vi "Teleop.vi"(0 "Call Context":T2, 1 "Match Info":T1={"Autonomous Elapsed Seconds"=0.0, "TeleOp Elapsed Seconds"=0.0, "Disabled Elapsed Seconds"=0.0, "Visited Autonomous"=FALSE, "Visited TeleOp"=FALSE, "Visited Disabled"=FALSE, "Autonomous Settings"={"Autonomous Style"=enum."Independent", "VI Refnum"=refnum}}) -> ()   [LabVIEW 2018]
doc: "This VI is called for each TeleOp packet received from the DS where the robot is not disabled. It is often used to read from the joysticks and update I/O or to update setpoints for timed control loops. It should complete and return within 20 milliseconds or it may miss DS packets."
uses:
  <vilib>/Rock Robotics/WPI/DriverStation/WPI_DriverStationDerivedRobotMode.ctl
  <vilib>/Rock Robotics/WPI/DriverStation/WPI_DriverStationMatch Info.ctl
  <vilib>/Rock Robotics/WPI/ThirdParty/Phoenix-LabVIEW/Motor Controller/Controls/CTRE_Phoenix_MotorControl_ControlMode.ctl
  <vilib>/Rock Robotics/WPI/Solenoid/WPI_SolenoidValue.ctl
  <vilib>/Rock Robotics/WPI/Utilities/WPI_GetSetVariantRefNum.vi
  <vilib>/Rock Robotics/Network Tables/NT Write Boolean Array.vi
  <vilib>/Rock Robotics/Network Tables/NT Write Numeric Array.vi
  <vilib>/Rock Robotics/Network Tables/NT Read Boolean.vi
  <vilib>/Rock Robotics/Network Tables/NT Read Number.vi
  <vilib>/Rock Robotics/WPI/Ultrasonic/WPI_SonarMB1010AnalogRefNum Registry Get.vi
  <vilib>/Rock Robotics/WPI/Ultrasonic/WPI_SonarMB1010AnalogGetRange.vi
  <vilib>/Rock Robotics/Network Tables/NT Write Number.vi
  <vilib>/Rock Robotics/WPI/Solenoid/WPI_SolenoidSetEnum.vi
panel:
  out "Distance":dbl
  out "FarRight":bool
  out "NearRight":bool
  out "NearLeft":bool
  out "FarLeft":bool
  out "Center":bool
  out "Compressor Running":bool
  out "Enabled":bool
  out "Sample Slider 0":dbl(slide) scale=0.0..5.0
  out "Sample Boolean 1":bool
  out "Sample Boolean 0":bool
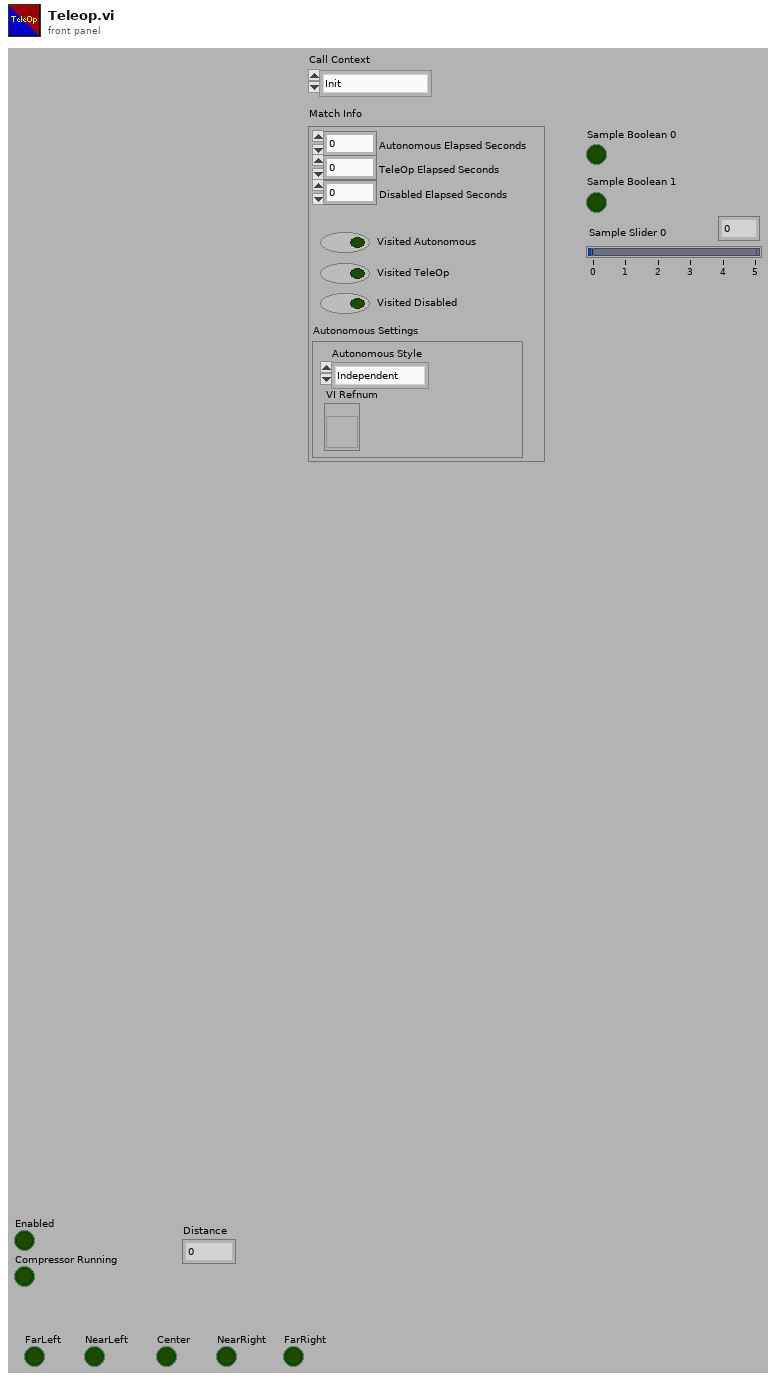
[diagram p1: front panel]
types:
  T1 = typedef "WPI_DriverStationMatch Info.ctl" = cluster{"Autonomous Elapsed Seconds":dbl, "TeleOp Elapsed Seconds":dbl, "Disabled Elapsed Seconds":dbl, "Visited Autonomous":bool, "Visited TeleOp":bool, "Visited Disabled":bool, "Autonomous Settings":cluster{"Autonomous Style":enum16{"Iterative", "Independent"}, "VI Refnum":refnum<vi>}}
  T2 = typedef "WPI_DriverStationDerivedRobotMode.ctl" = enum16{"Init", "Execute", "Stop"}
  T3 = typedef "WPI_JoystickDevRef.ctl" = cluster{"Device":T4}
  T4 = typedef "WPI_JoystickDeviceEnum.ctl" = enum16{"USB 0", "USB 1", "USB 2", "USB 3", "USB 4", "USB 5"}
  T5 = typedef "WPI_DigitalInputDevRef.ctl" = cluster{"DevStatus":errorcluster, "DIO Channel":T6}
  T6 = typedef "FPGA_DIOChannel.ctl" = enum8{"DIO 0", "DIO 1", "DIO 2", "DIO 3", "DIO 4", "DIO 5", "DIO 6", "DIO 7", "DIO 8", "DIO 9", "DIO MXP 0", "DIO MXP 1", "DIO MXP 2", "DIO MXP 3", "DIO MXP 4", "DIO MXP 5", "DIO MXP 6", "DIO MXP 7", "DIO MXP 8", "DIO MXP 9", "DIO MXP 10", "DIO MXP 11", "DIO MXP 12", "DIO MXP 13", "DIO MXP 14", "DIO MXP 15", "SPI Port CS1", "SPI Port CS2", "SPI Port CS3", "SPI Port MISO", "SPI Port MOSI", "Invalid"}
  T7 = typedef "CTRE_Phoenix_MotorControl_ControlMode.ctl" = u16
  T8 = typedef "WPI_MotorControlDeviceRef.ctl" = cluster{"DeviceStatus":errorcluster, "Type":T9, "PWM":cluster{"PWM Channel":T10, "DeadBand":T11}, "CAN":cluster{"Device Number":u8, "SetOutput VI Ref":variant, "GetOutput VI Ref":variant, "Enable VI Ref":variant, "Disable VI Ref":variant, "Data":variant}, "Invert":bool, "DIO PWM":cluster{"PWM \"Enable\" Channel":T10, "DIOChannel":T6, "PWM Rate":dbl}}
  T9 = typedef "WPI_MotorControlType.ctl" = enum16{"PWM", "CAN", "DIO PWM"}
  T10 = typedef "FPGA_DIOPWMChannel.ctl" = enum8{"PWM 0", "PWM 1", "PWM 2", "PWM 3", "PWM 4", "PWM 5", "PWM 6", "PWM 7", "PWM 8", "PWM 9", "PWM MXP 0", "PWM MXP 1", "PWM MXP 2", "PWM MXP 3", "PWM MXP 4", "PWM MXP 5", "PWM MXP 6", "PWM MXP 7", "PWM MXP 8", "PWM MXP 9", "Invalid"}
  T11 = typedef "WPI_PWMDeadband.ctl" = cluster{"Name":string, "maxPositivePwm":i32, "minPositivePwm":i32, "centerPwm":i32, "maxNegativePwm":i32, "minNegativePwm":i32, "angularRange":u16}
  T12 = typedef "WPI_SolenoidValue.ctl" = enum16{"Off", "On", "Forward", "Reverse"}
  T13 = typedef "WPI_SolenoidDevRef.ctl" = cluster{"DevStatus":errorcluster, "Pneumatics Control Module":u8, "Forward Solenoid Channel":T14, "Reverse Solenoid Channel":T14}
  T14 = typedef "WPI_SolenoidChannel.ctl" = enum8{"Solenoid 0", "Solenoid 1", "Solenoid 2", "Solenoid 3", "Solenoid 4", "Solenoid 5", "Solenoid 6", "Solenoid 7", "Invalid"}
  T15 = typedef "WPI_SonarMB1010AnalogDeviceRef.ctl" = cluster{"AIDeviceRef":T16, "Scaling factor (V/in)":dbl, "Average Bits":u8}
  T16 = typedef "WPI_AnalogChannelDevRef.ctl" = cluster{"DevStatus":errorcluster, "Analog Channel":T17}
  T17 = typedef "FPGA_AIChannel.ctl" = enum8{"AI 0", "AI 1", "AI 2", "AI 3", "AI MXP 0", "AI MXP 1", "AI MXP 2", "AI MXP 3", "Invalid"}
  T18 = typedef "WPI_CompressorDevRef.ctl" = cluster{"DevStatus":errorcluster, "Pneumatics Control Module":u8}
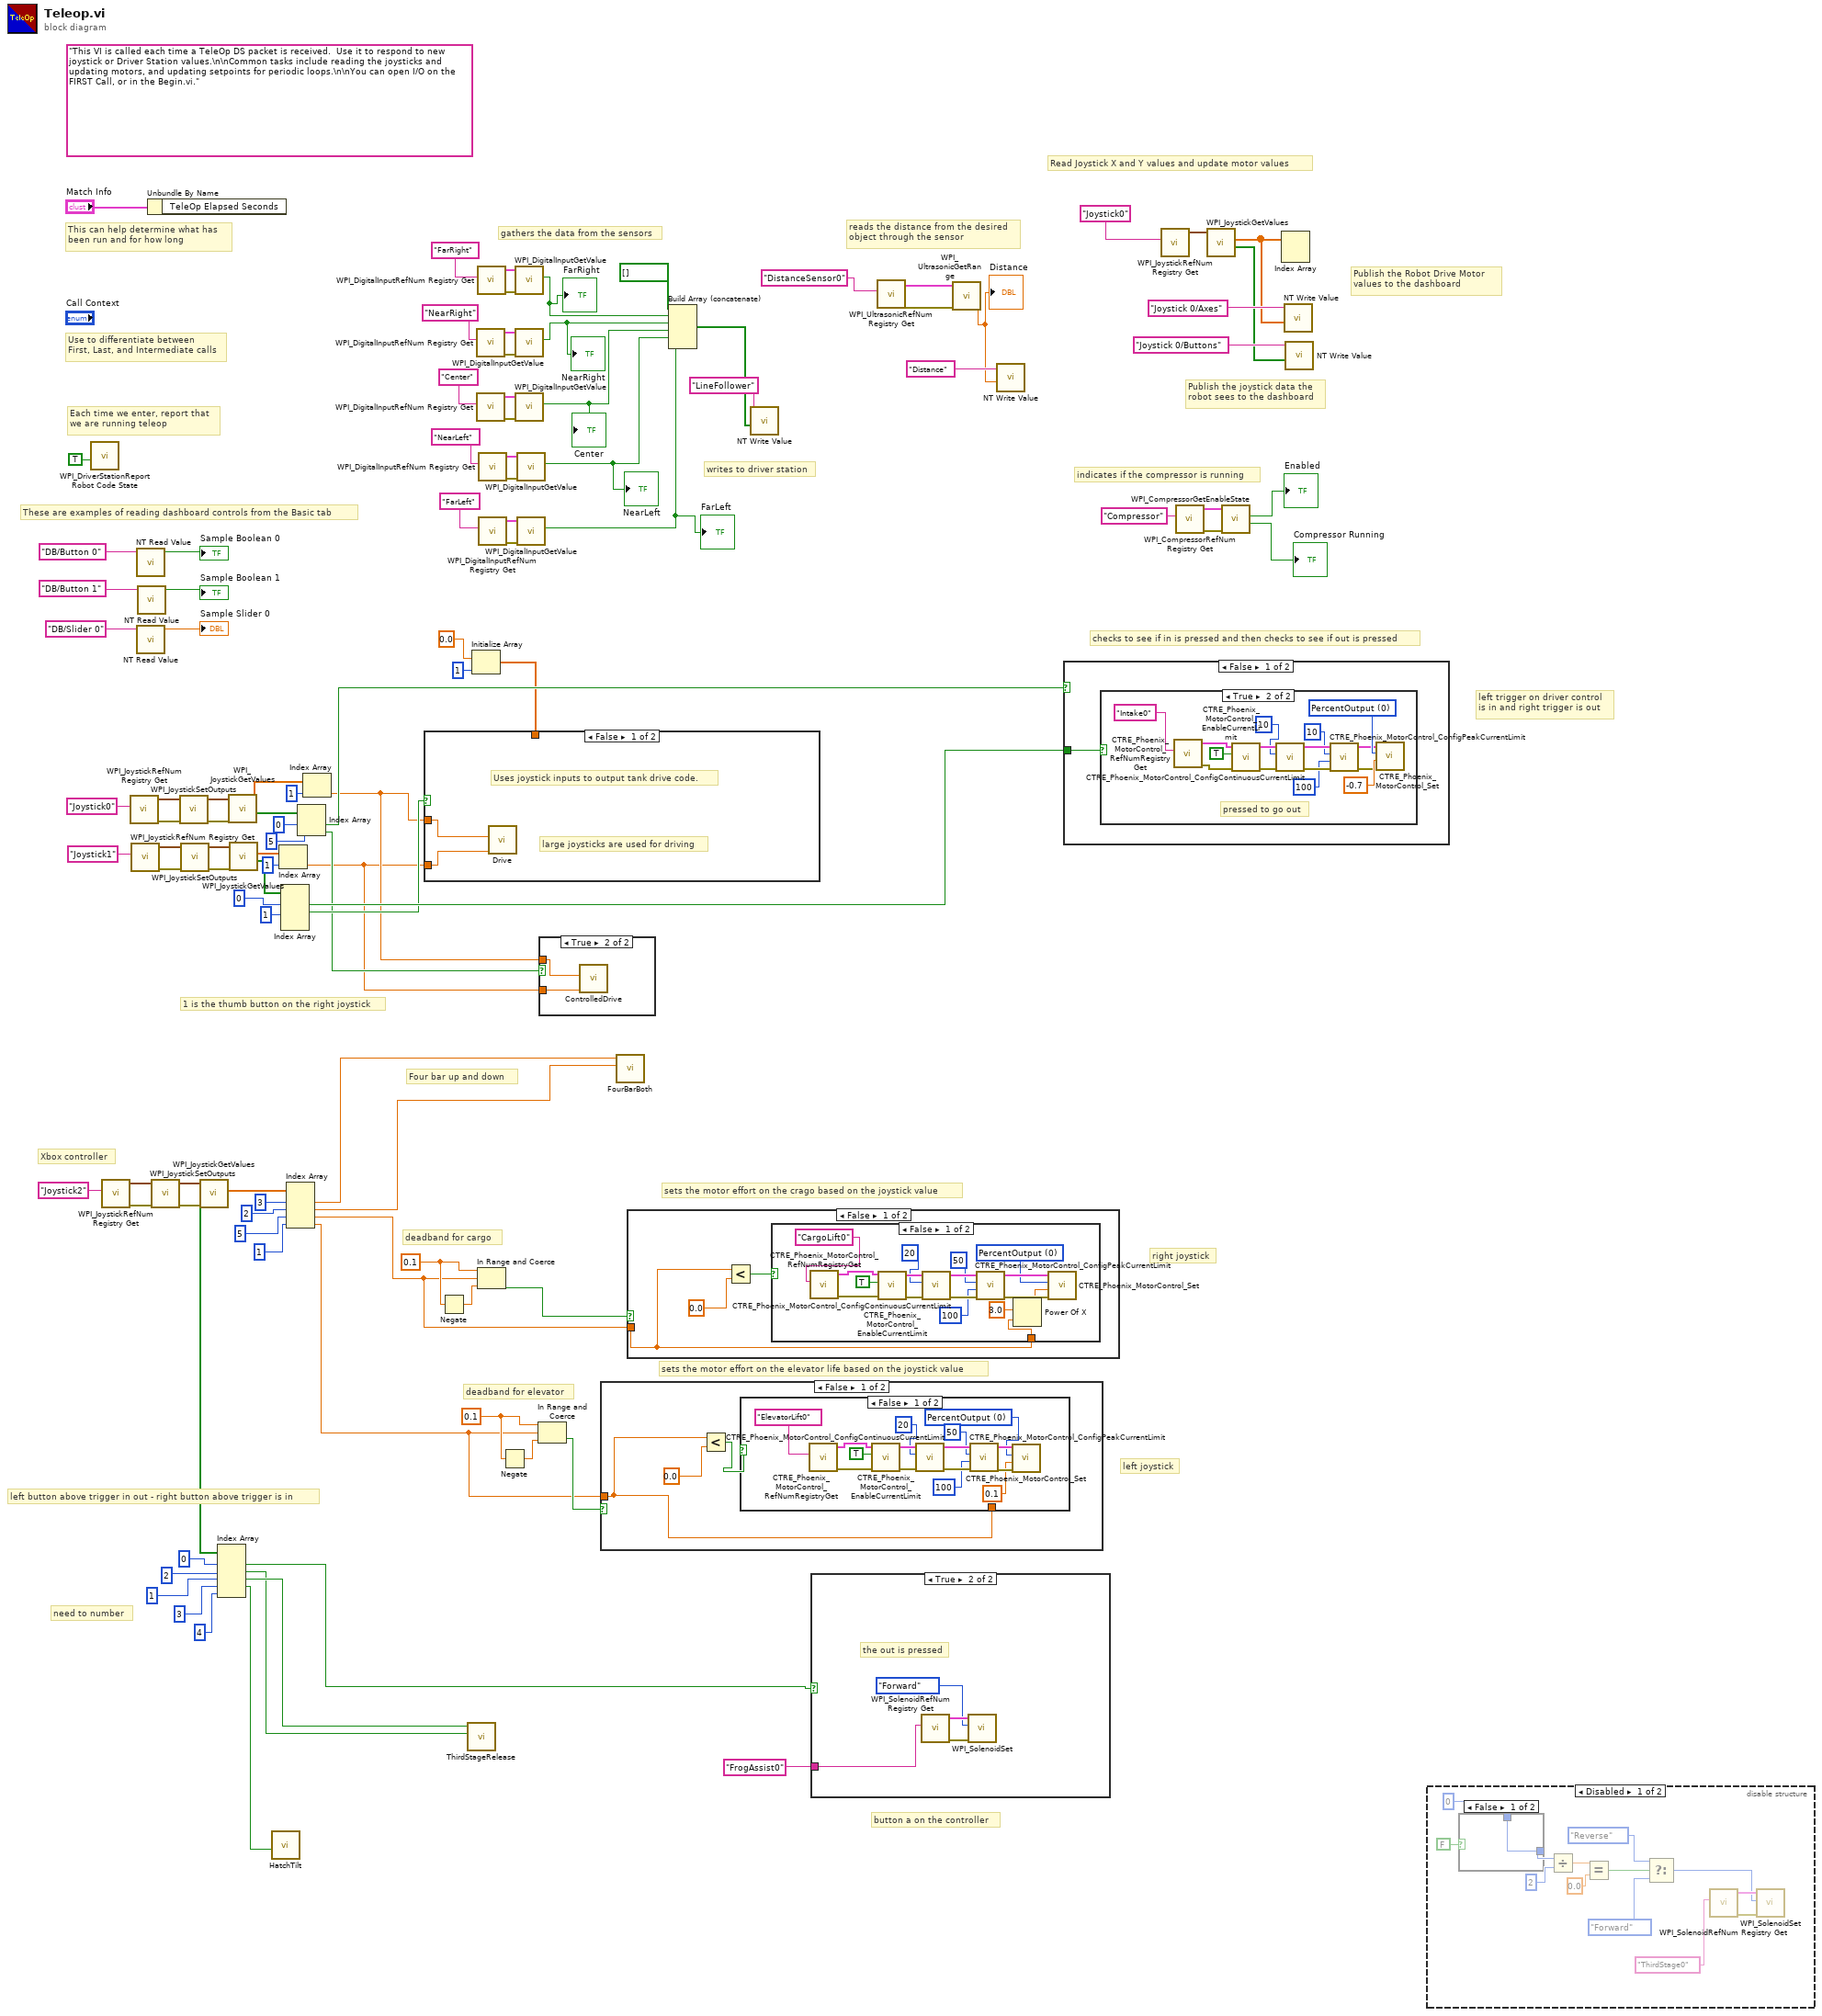
[diagram p0: block diagram]
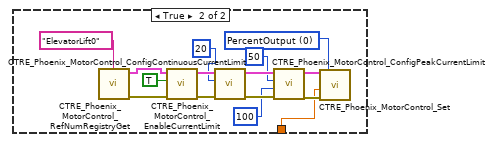
[diagram p3: hidden frame]
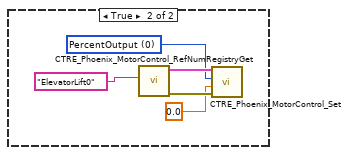
[diagram p4: hidden frame]
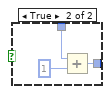
[diagram p5: hidden frame]
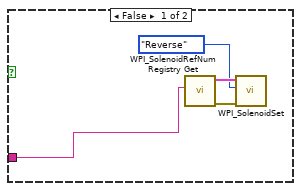
[diagram p7: hidden frame]
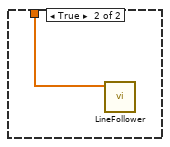
[diagram p8: hidden frame]
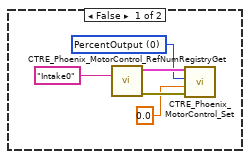
[diagram p9: hidden frame]
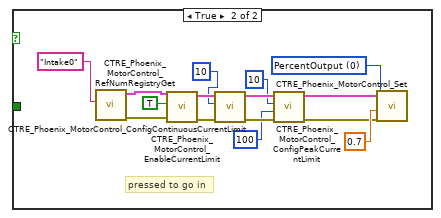
[diagram p10: hidden frame]
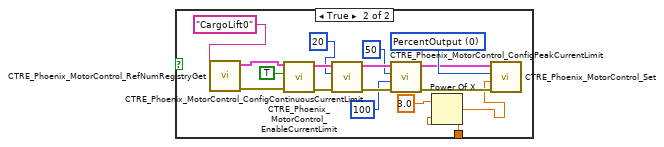
[diagram p11: hidden frame]
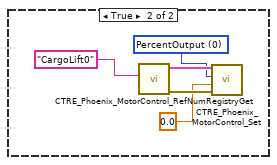
[diagram p12: hidden frame]
diagram:
  w52 = 0.1 ("upper limit")
  w55 = 0.1 ("upper limit")
  (unwired) "This VI is called each time a TeleOp DS packet is received.  Use it to respond to new joystick or Driver Station values.\n\nCommon tasks include reading the joysticks and updating motors, and updating setpoints for periodic loops.\n\nYou can open I/O on the FIRST Call, or in the Begin.vi."
  # "left joystick"
  # "sets the motor effort on the elevator life based on the joystick value"
  # "reads the distance from the desired\nobject through the sensor"
  # "button a on the controller"
  # "gathers the data from the sensors"
  # "writes to driver station"
  # "1 is the thumb button on the right joystick"
  # "left trigger on driver control\nis in and right trigger is out"
  # "checks to see if in is pressed and then checks to see if out is pressed"
  # "right joystick"
  # "deadband for elevator"
  # "deadband for cargo"
  # "sets the motor effort on the crago based on the joystick value"
  # "Four bar up and down"
  # "indicates if the compressor is running"
  # "need to number"
  # "left button above trigger in out - right button above trigger is in"
  # "Xbox controller"
  # "These are examples of reading dashboard controls from the Basic tab"
  # "Publish the Robot Drive Motor\nvalues to the dashboard"
  # "Publish the joystick data the\nrobot sees to the dashboard"
  # "Each time we enter, report that\nwe are running teleop"
  # "Use to differentiate between\nFirst, Last, and Intermediate calls"
  # "This can help determine what has\nbeen run and for how long"
  # "Read Joystick X and Y values and update motor values"
  n1 = call <vilib>:"WPI_DriverStationReport Robot Code State.vi"("TeleOp"=TRUE ("Autonomous")) -> ()  [unwired: 10 in, 1 out]
  n2 = call <vilib>:"WPI_JoystickRefNum Registry Get.vi"("refnum name"="Joystick2") -> ("error out"=w76:errorcluster, "JoystickDevRef"=w78:T3)  [unwired: 1 in, 8 out]
  n3 = call <vilib>:"WPI_JoystickRefNum Registry Get.vi"("refnum name"="Joystick0") -> ("error out"=w89:errorcluster, "JoystickDevRef"=w91:T3)  [unwired: 1 in, 8 out]
  n4 = call <vilib>:"WPI_JoystickRefNum Registry Get.vi"("refnum name"="Joystick1") -> ("error out"=w86:errorcluster, "JoystickDevRef"=w84:T3)  [unwired: 1 in, 8 out]
  n5 = call-poly <vilib>:"NT Read Value.vi"("Name"="DB/Button 0" ("refnum name")) -> ("Boolean"=→"Sample Boolean 0":bool)  [unwired: 9 in, 1 out]
  n6 = call-poly <vilib>:"NT Read Value.vi"("Name"="DB/Slider 0" ("refnum name")) -> ("Numeric"=→"Sample Slider 0":dbl)  [unwired: 9 in, 1 out]
  n7 = call-poly <vilib>:"NT Read Value.vi"("Name"="DB/Button 1" ("refnum name")) -> ("Boolean"=→"Sample Boolean 1":bool)  [unwired: 9 in, 1 out]
  n8 = Unbundle By Name("Match Info") -> ()  [unwired: 1 out]
  n9 = call <vilib>:"WPI_JoystickSetOutputs.vi"("error in (no error)"=w76, "JoystickDevRef"=w78) -> ("error out"=w75:errorcluster, "JoystickDevRef"=w77:T3)  [unwired: 8 in]
  n10 = call <vilib>:"WPI_JoystickSetOutputs.vi"("error in (no error)"=w89, "JoystickDevRef"=w91) -> ("error out"=w88:errorcluster, "JoystickDevRef"=w90:T3)  [unwired: 8 in]
  n11 = call <vilib>:"WPI_JoystickSetOutputs.vi"("error in (no error)"=w86, "JoystickDevRef"=w84) -> ("error out"=w87:errorcluster, "JoystickDevRef"=w85:T3)  [unwired: 8 in]
  n12 = call <vilib>:"WPI_JoystickGetValues.vi"("error in (no error)"=w75, "JoystickDevRef"=w77) -> ("Buttons"=w74:bool[], "Axes"=w71:dbl[])  [unwired: 5 in, 3 out]
  n13 = Index Array(array=w74, index #1=0 ("index"), index #2=2 ("index"), index #3=1 ("index"), index #4=3 ("index"), index #5=4 ("index")) -> (element #1=w16:bool, element #2=w8:bool, element #3=w9:bool, element #4=w10:bool)  [unwired: 1 out]
  n14 = call <vilib>:"WPI_JoystickGetValues.vi"("error in (no error)"=w88, "JoystickDevRef"=w90) -> ("Buttons"=w80:bool[], "Axes"=w93:dbl[])  [unwired: 5 in, 3 out]
  n15 = call <vilib>:"WPI_JoystickGetValues.vi"("error in (no error)"=w87, "JoystickDevRef"=w85) -> ("Buttons"=w65:bool[], "Axes"=w82:dbl[])  [unwired: 5 in, 3 out]
  n16 = call "HatchTilt.vi"("Boolean"=w10) -> ()  [unwired: 11 in]
  n17 = Index Array(array=w82, index=1) -> (element=w1:dbl)
  n18 = Index Array(array=w65, index #1=0 ("index"), index #2=1 ("index")) -> (element #1=w46:bool, element #2=w21:bool)  [unwired: 2 in, 2 out]
  n19 = Index Array(array=w71, index #1=3 ("index"), index #2=2 ("index"), index #3=5 ("index"), index #4=1 ("index")) -> (element #1=w6:dbl, element #2=w5:dbl, element #3=w54:dbl, element #4=w50:dbl)
  n20 = Index Array(array=w80, index #1=0 ("index"), index #2=5 ("index")) -> (element #1=w47:bool, element #2=w3:bool)
  n21 = Index Array(array=w93, index=1) -> (element=w2:dbl)
  n22 = Negate(x=w55) -> (-x=w57:dbl)
  n23 = call "ThirdStageRelease.vi"("In"=w8, "Out"=w9) -> ()  [unwired: 10 in]
  n24 = Initialize Array(0.0 ("element"), 1 ("dimension size")) -> (w18:dbl[])
  n25 = case shown="False" w21 {
    tunnel: w2 -> [w109 _]
    tunnel: w1 -> [w108 _]
    tunnel: w18 -> [_ w110]
    frame False {
      # "large joysticks are used for driving"
      # "Uses joystick inputs to output tank drive code."
      n26 = call "Drive.vi"("Drive R"=w108, "Drive L"=w109) -> ()  [unwired: 10 in]
    }
    frame True {
      n27 = call "LineFollower.vi"("LastNumArray"=w110) -> ()  [unwired: 11 in]
    }
  }
  n28 = call <vilib>:"WPI_DigitalInputRefNum Registry Get.vi"("refnum name"="NearRight") -> ("error out"=w41:errorcluster, "DigitalInputDevRef"=w40:T5)  [unwired: 9 in]
  n29 = call <vilib>:"WPI_DigitalInputRefNum Registry Get.vi"("refnum name"="Center") -> ("error out"=w38:errorcluster, "DigitalInputDevRef"=w37:T5)  [unwired: 9 in]
  n30 = call <vilib>:"WPI_DigitalInputRefNum Registry Get.vi"("refnum name"="FarRight") -> ("error out"=w44:errorcluster, "DigitalInputDevRef"=w43:T5)  [unwired: 9 in]
  n31 = In Range and Coerce(upper limit=w55, x=w54, lower limit=w57) -> (In Range?=w56:bool)  [unwired: 1 out]
  n32 = call <vilib>:"WPI_DigitalInputRefNum Registry Get.vi"("refnum name"="NearLeft") -> ("error out"=w35:errorcluster, "DigitalInputDevRef"=w34:T5)  [unwired: 9 in]
  n33 = call <vilib>:"WPI_DigitalInputRefNum Registry Get.vi"("refnum name"="FarLeft") -> ("error out"=w32:errorcluster, "DigitalInputDevRef"=w31:T5)  [unwired: 9 in]
  n34 = Negate(x=w52) -> (-x=w53:dbl)
  n35 = call <vilib>:"WPI_DigitalInputGetValue.vi"("error in (no error)"=w44, "DigitalInputDevRef"=w43) -> ("Value"=w28:bool)  [unwired: 7 in, 2 out]
  "FarRight" <- w28
  n36 = call <vilib>:"WPI_DigitalInputGetValue.vi"("error in (no error)"=w41, "DigitalInputDevRef"=w40) -> ("Value"=w27:bool)  [unwired: 7 in, 2 out]
  "NearRight" <- w27
  n37 = call <vilib>:"WPI_DigitalInputGetValue.vi"("error in (no error)"=w38, "DigitalInputDevRef"=w37) -> ("Value"=w29:bool)  [unwired: 7 in, 2 out]
  "Center" <- w29
  n38 = call <vilib>:"WPI_DigitalInputGetValue.vi"("error in (no error)"=w35, "DigitalInputDevRef"=w34) -> ("Value"=w26:bool)  [unwired: 7 in, 2 out]
  "NearLeft" <- w26
  n39 = call <vilib>:"WPI_DigitalInputGetValue.vi"("error in (no error)"=w32, "DigitalInputDevRef"=w31) -> ("Value"=w25:bool)  [unwired: 7 in, 2 out]
  "FarLeft" <- w25
  n40 = In Range and Coerce(upper limit=w52, x=w50, lower limit=w53) -> (In Range?=w51:bool)  [unwired: 1 out]
  n41 = case shown="True" w3 {
    tunnel: w2 -> [_ w112]
    tunnel: w1 -> [_ w111]
    frame False {
    }
    frame True {
      n42 = call "ControlledDrive.vi"("Drive R"=w111, "Drive L"=w112) -> ()  [unwired: 10 in]
    }
  }
  n43 = case shown="False" w51 {
    tunnel: w50 -> [w113 _]
    frame False {
      n44 = Less?(x=w113, y=0.0) -> (x < y?=w115:bool)
      n45 = case shown="False" w115 {
        tunnel: w113 -> [_ w131]
        frame False {
          w122 = T7 0 items=["PercentOutput"=0, "Position"=1, "Velocity"=2, "Current"=3, "Follower"=5, "MotionProfile"=6, "MotionMagic"=7, "MotionMagicArc"=8, "MotionProfileArc"=10, "Disabled"=15] ("Control Mode")
          n46 = call <vilib>:"CTRE_Phoenix_MotorControl_RefNumRegistryGet.vi"("refnum name"="ElevatorLift0") -> ("error out"=w128:errorcluster, "PhoenixMotorControlDevRef"=w127:T8)  [unwired: 9 in]
          n47 = call <vilib>:"CTRE_Phoenix_MotorControl_EnableCurrentLimit.vi"("error in (no error)"=w128, "Enable Current Limit?"=TRUE, "PhoenixMotorControlDevRef"=w127) -> ("error out"=w123:errorcluster, "PhoenixMotorControlDevRef"=w124:T8)  [unwired: 7 in]
          n48 = call <vilib>:"CTRE_Phoenix_MotorControl_ConfigContinuousCurrentLimit.vi"("error in (no error)"=w123, "Continuous Current Limit (Amps)"=20, "PhoenixMotorControlDevRef"=w124) -> ("error out"=w126:errorcluster, "PhoenixMotorControlDevRef"=w125:T8)  [unwired: 7 in]
          n49 = call <vilib>:"CTRE_Phoenix_MotorControl_ConfigPeakCurrentLimit.vi"("error in (no error)"=w126, "Peak Current Maximum Duration (ms)"=100, "Peak Current (Amps)"=50, "PhoenixMotorControlDevRef"=w125) -> ("error out"=w130:errorcluster, "PhoenixMotorControlDevRef"=w129:T8)  [unwired: 6 in]
          n50 = call <vilib>:"CTRE_Phoenix_MotorControl_Set.vi"("error in (no error)"=w130, "Output"=0.1, "Control Mode"=w122, "PhoenixMotorControlDevRef"=w129) -> ()  [unwired: 6 in, 2 out]
        }
        frame True {
          w145 = T7 0 items=["PercentOutput"=0, "Position"=1, "Velocity"=2, "Current"=3, "Follower"=5, "MotionProfile"=6, "MotionMagic"=7, "MotionMagicArc"=8, "MotionProfileArc"=10, "Disabled"=15] ("Control Mode")
          n51 = call <vilib>:"CTRE_Phoenix_MotorControl_RefNumRegistryGet.vi"("refnum name"="ElevatorLift0") -> ("error out"=w135:errorcluster, "PhoenixMotorControlDevRef"=w136:T8)  [unwired: 9 in]
          n52 = call <vilib>:"CTRE_Phoenix_MotorControl_EnableCurrentLimit.vi"("error in (no error)"=w135, "Enable Current Limit?"=TRUE, "PhoenixMotorControlDevRef"=w136) -> ("error out"=w142:errorcluster, "PhoenixMotorControlDevRef"=w141:T8)  [unwired: 7 in]
          n53 = call <vilib>:"CTRE_Phoenix_MotorControl_ConfigContinuousCurrentLimit.vi"("error in (no error)"=w142, "Continuous Current Limit (Amps)"=20, "PhoenixMotorControlDevRef"=w141) -> ("error out"=w139:errorcluster, "PhoenixMotorControlDevRef"=w140:T8)  [unwired: 7 in]
          n54 = call <vilib>:"CTRE_Phoenix_MotorControl_ConfigPeakCurrentLimit.vi"("error in (no error)"=w139, "Peak Current Maximum Duration (ms)"=100, "Peak Current (Amps)"=50, "PhoenixMotorControlDevRef"=w140) -> ("error out"=w133:errorcluster, "PhoenixMotorControlDevRef"=w134:T8)  [unwired: 6 in]
          n55 = call <vilib>:"CTRE_Phoenix_MotorControl_Set.vi"("error in (no error)"=w133, "Output"=w131, "Control Mode"=w145, "PhoenixMotorControlDevRef"=w134) -> ()  [unwired: 6 in, 2 out]
        }
      }
    }
    frame True {
      w146 = T7 0 items=["PercentOutput"=0, "Position"=1, "Velocity"=2, "Current"=3, "Follower"=5, "MotionProfile"=6, "MotionMagic"=7, "MotionMagicArc"=8, "MotionProfileArc"=10, "Disabled"=15] ("Control Mode")
      n56 = call <vilib>:"CTRE_Phoenix_MotorControl_RefNumRegistryGet.vi"("refnum name"="ElevatorLift0") -> ("error out"=w150:errorcluster, "PhoenixMotorControlDevRef"=w149:T8)  [unwired: 9 in]
      n57 = call <vilib>:"CTRE_Phoenix_MotorControl_Set.vi"("error in (no error)"=w150, "Output"=0.0, "Control Mode"=w146, "PhoenixMotorControlDevRef"=w149) -> ()  [unwired: 6 in, 2 out]
    }
  }
  n58 = call "FourBarBoth.vi"("Down"=w5, "Up"=w6) -> ()  [unwired: 10 in]
  n59 = case shown="False" w56 {
    tunnel: w54 -> [w151 _]
    frame False {
      n60 = Less?(x=w151, y=0.0) -> (x < y?=w152:bool)
      n61 = case shown="False" w152 {
        tunnel: w151 -> [w155 w171]
        frame False {
          w162 = T7 0 items=["PercentOutput"=0, "Position"=1, "Velocity"=2, "Current"=3, "Follower"=5, "MotionProfile"=6, "MotionMagic"=7, "MotionMagicArc"=8, "MotionProfileArc"=10, "Disabled"=15] ("Control Mode")
          n62 = call <vilib>:"CTRE_Phoenix_MotorControl_RefNumRegistryGet.vi"("refnum name"="CargoLift0") -> ("error out"=w168:errorcluster, "PhoenixMotorControlDevRef"=w167:T8)  [unwired: 9 in]
          n63 = call <vilib>:"CTRE_Phoenix_MotorControl_EnableCurrentLimit.vi"("error in (no error)"=w168, "Enable Current Limit?"=TRUE, "PhoenixMotorControlDevRef"=w167) -> ("error out"=w163:errorcluster, "PhoenixMotorControlDevRef"=w164:T8)  [unwired: 7 in]
          n64 = call <vilib>:"CTRE_Phoenix_MotorControl_ConfigContinuousCurrentLimit.vi"("error in (no error)"=w163, "Continuous Current Limit (Amps)"=20, "PhoenixMotorControlDevRef"=w164) -> ("error out"=w166:errorcluster, "PhoenixMotorControlDevRef"=w165:T8)  [unwired: 7 in]
          n65 = call <vilib>:"CTRE_Phoenix_MotorControl_ConfigPeakCurrentLimit.vi"("error in (no error)"=w166, "Peak Current Maximum Duration (ms)"=100, "Peak Current (Amps)"=50, "PhoenixMotorControlDevRef"=w165) -> ("error out"=w170:errorcluster, "PhoenixMotorControlDevRef"=w169:T8)  [unwired: 6 in]
          n66 = Power Of X(1:w155, 2:3.0 ("y")) -> (0:w154:dbl)
          n67 = call <vilib>:"CTRE_Phoenix_MotorControl_Set.vi"("error in (no error)"=w170, "Output"=w154, "Control Mode"=w162, "PhoenixMotorControlDevRef"=w169) -> ()  [unwired: 6 in, 2 out]
        }
        frame True {
          w187 = T7 0 items=["PercentOutput"=0, "Position"=1, "Velocity"=2, "Current"=3, "Follower"=5, "MotionProfile"=6, "MotionMagic"=7, "MotionMagicArc"=8, "MotionProfileArc"=10, "Disabled"=15] ("Control Mode")
          n68 = call <vilib>:"CTRE_Phoenix_MotorControl_RefNumRegistryGet.vi"("refnum name"="CargoLift0") -> ("error out"=w178:errorcluster, "PhoenixMotorControlDevRef"=w179:T8)  [unwired: 9 in]
          n69 = call <vilib>:"CTRE_Phoenix_MotorControl_EnableCurrentLimit.vi"("error in (no error)"=w178, "Enable Current Limit?"=TRUE, "PhoenixMotorControlDevRef"=w179) -> ("error out"=w185:errorcluster, "PhoenixMotorControlDevRef"=w184:T8)  [unwired: 7 in]
          n70 = call <vilib>:"CTRE_Phoenix_MotorControl_ConfigContinuousCurrentLimit.vi"("error in (no error)"=w185, "Continuous Current Limit (Amps)"=20, "PhoenixMotorControlDevRef"=w184) -> ("error out"=w182:errorcluster, "PhoenixMotorControlDevRef"=w183:T8)  [unwired: 7 in]
          n71 = call <vilib>:"CTRE_Phoenix_MotorControl_ConfigPeakCurrentLimit.vi"("error in (no error)"=w182, "Peak Current Maximum Duration (ms)"=100, "Peak Current (Amps)"=50, "PhoenixMotorControlDevRef"=w183) -> ("error out"=w176:errorcluster, "PhoenixMotorControlDevRef"=w177:T8)  [unwired: 6 in]
          n72 = Power Of X(1:w171, 2:3.0 ("y")) -> (0:w173:dbl)
          n73 = call <vilib>:"CTRE_Phoenix_MotorControl_Set.vi"("error in (no error)"=w176, "Output"=w173, "Control Mode"=w187, "PhoenixMotorControlDevRef"=w177) -> ()  [unwired: 6 in, 2 out]
        }
      }
    }
    frame True {
      w189 = T7 0 items=["PercentOutput"=0, "Position"=1, "Velocity"=2, "Current"=3, "Follower"=5, "MotionProfile"=6, "MotionMagic"=7, "MotionMagicArc"=8, "MotionProfileArc"=10, "Disabled"=15] ("Control Mode")
      n74 = call <vilib>:"CTRE_Phoenix_MotorControl_RefNumRegistryGet.vi"("refnum name"="CargoLift0") -> ("error out"=w192:errorcluster, "PhoenixMotorControlDevRef"=w191:T8)  [unwired: 9 in]
      n75 = call <vilib>:"CTRE_Phoenix_MotorControl_Set.vi"("error in (no error)"=w192, "Output"=0.0, "Control Mode"=w189, "PhoenixMotorControlDevRef"=w191) -> ()  [unwired: 6 in, 2 out]
    }
  }
  n76 = Build Array (concatenate)(bool[] [] ("array"), w28, w27, w29, w26, w25) -> (w24:bool[])
  n77 = call-poly <vilib>:"NT Write Value.vi"("Boolean Array"=w24, "Name"="LineFollower") -> ()  [unwired: 9 in, 1 out]
  n78 = case shown="True" w16 {
    tunnel: "FrogAssist0" ("refnum name") -> [w193 w197]
    frame False {
      n79 = call <vilib>:"WPI_SolenoidRefNum Registry Get.vi"("refnum name"=w193) -> ("error out"=w196:errorcluster, "SolenoidDevRef"=w195:T13)  [unwired: 9 in]
      n80 = call-poly <vilib>:"WPI_SolenoidSet.vi"("error in (no error)"=w196, "Value"=WPI_SolenoidValue."Reverse", "SolenoidDevRef"=w195) -> ()  [unwired: 7 in, 2 out]
    }
    frame True {
      # "the out is pressed"
      n81 = call <vilib>:"WPI_SolenoidRefNum Registry Get.vi"("refnum name"=w197) -> ("error out"=w199:errorcluster, "SolenoidDevRef"=w200:T13)  [unwired: 9 in]
      n82 = call-poly <vilib>:"WPI_SolenoidSet.vi"("error in (no error)"=w199, "Value"=WPI_SolenoidValue."Forward", "SolenoidDevRef"=w200) -> ()  [unwired: 7 in, 2 out]
    }
  }
  n83 = call-poly <vilib>:"WPI_UltrasonicRefNum Registry Get.vi"("refnum name"="DistanceSensor0") -> ("error out"=w14:errorcluster, "SonarMB1010AnalogDevRef"=w15:T15)  [unwired: 9 in]
  n84 = call-poly <vilib>:"WPI_UltrasonicGetRange.vi"("error in"=w14, "SonarMB1010AnalogDevRef"=w15) -> ("Distance"=w11:dbl)  [unwired: 7 in, 2 out]
  "Distance" <- w11
  n85 = call-poly <vilib>:"NT Write Value.vi"("Numeric"=w11, "Name"="Distance") -> ()  [unwired: 9 in, 1 out]
  n86 = case shown="False" w47 {
    tunnel: w46 -> [w201 _]
    frame False {
      n87 = case shown="True" w201 {
        frame False {
          w203 = T7 0 items=["PercentOutput"=0, "Position"=1, "Velocity"=2, "Current"=3, "Follower"=5, "MotionProfile"=6, "MotionMagic"=7, "MotionProfileArc"=10, "Disabled"=15] ("Control Mode")
          n88 = call <vilib>:"CTRE_Phoenix_MotorControl_RefNumRegistryGet.vi"("refnum name"="Intake0") -> ("error out"=w205:errorcluster, "PhoenixMotorControlDevRef"=w206:T8)  [unwired: 9 in]
          n89 = call <vilib>:"CTRE_Phoenix_MotorControl_Set.vi"("error in (no error)"=w205, "Output"=0.0, "Control Mode"=w203, "PhoenixMotorControlDevRef"=w206) -> ()  [unwired: 6 in, 2 out]
        }
        frame True {
          w220 = T7 0 items=["PercentOutput"=0, "Position"=1, "Velocity"=2, "Current"=3, "Follower"=5, "MotionProfile"=6, "MotionMagic"=7, "MotionProfileArc"=10, "Disabled"=15] ("Control Mode")
          # "pressed to go out"
          n90 = call <vilib>:"CTRE_Phoenix_MotorControl_RefNumRegistryGet.vi"("refnum name"="Intake0") -> ("error out"=w210:errorcluster, "PhoenixMotorControlDevRef"=w211:T8)  [unwired: 9 in]
          n91 = call <vilib>:"CTRE_Phoenix_MotorControl_EnableCurrentLimit.vi"("error in (no error)"=w210, "Enable Current Limit?"=TRUE, "PhoenixMotorControlDevRef"=w211) -> ("error out"=w217:errorcluster, "PhoenixMotorControlDevRef"=w216:T8)  [unwired: 7 in]
          n92 = call <vilib>:"CTRE_Phoenix_MotorControl_ConfigContinuousCurrentLimit.vi"("error in (no error)"=w217, "Continuous Current Limit (Amps)"=10, "PhoenixMotorControlDevRef"=w216) -> ("error out"=w214:errorcluster, "PhoenixMotorControlDevRef"=w215:T8)  [unwired: 7 in]
          n93 = call <vilib>:"CTRE_Phoenix_MotorControl_ConfigPeakCurrentLimit.vi"("error in (no error)"=w214, "Peak Current Maximum Duration (ms)"=100, "Peak Current (Amps)"=10, "PhoenixMotorControlDevRef"=w215) -> ("error out"=w208:errorcluster, "PhoenixMotorControlDevRef"=w209:T8)  [unwired: 6 in]
          n94 = call <vilib>:"CTRE_Phoenix_MotorControl_Set.vi"("error in (no error)"=w208, "Output"=-0.7, "Control Mode"=w220, "PhoenixMotorControlDevRef"=w209) -> ()  [unwired: 6 in, 2 out]
        }
      }
    }
    frame True {
      w234 = T7 0 items=["PercentOutput"=0, "Position"=1, "Velocity"=2, "Current"=3, "Follower"=5, "MotionProfile"=6, "MotionMagic"=7, "MotionProfileArc"=10, "Disabled"=15] ("Control Mode")
      # "pressed to go in"
      n95 = call <vilib>:"CTRE_Phoenix_MotorControl_RefNumRegistryGet.vi"("refnum name"="Intake0") -> ("error out"=w224:errorcluster, "PhoenixMotorControlDevRef"=w223:T8)  [unwired: 9 in]
      n96 = call <vilib>:"CTRE_Phoenix_MotorControl_EnableCurrentLimit.vi"("error in (no error)"=w224, "Enable Current Limit?"=TRUE, "PhoenixMotorControlDevRef"=w223) -> ("error out"=w232:errorcluster, "PhoenixMotorControlDevRef"=w231:T8)  [unwired: 7 in]
      n97 = call <vilib>:"CTRE_Phoenix_MotorControl_ConfigContinuousCurrentLimit.vi"("error in (no error)"=w232, "Continuous Current Limit (Amps)"=10, "PhoenixMotorControlDevRef"=w231) -> ("error out"=w229:errorcluster, "PhoenixMotorControlDevRef"=w230:T8)  [unwired: 7 in]
      n98 = call <vilib>:"CTRE_Phoenix_MotorControl_ConfigPeakCurrentLimit.vi"("error in (no error)"=w229, "Peak Current Maximum Duration (ms)"=100, "Peak Current (Amps)"=10, "PhoenixMotorControlDevRef"=w230) -> ("error out"=w225:errorcluster, "PhoenixMotorControlDevRef"=w226:T8)  [unwired: 6 in]
      n99 = call <vilib>:"CTRE_Phoenix_MotorControl_Set.vi"("error in (no error)"=w225, "Output"=0.7, "Control Mode"=w234, "PhoenixMotorControlDevRef"=w226) -> ()  [unwired: 6 in, 2 out]
    }
  }
  n100 = call <vilib>:"WPI_JoystickRefNum Registry Get.vi"("refnum name"="Joystick0") -> ("JoystickDevRef"=w105:T3)  [unwired: 1 in, 9 out]
  n101 = call <vilib>:"WPI_CompressorRefNum Registry Get.vi"("refnum name"="Compressor") -> ("error out"=w70:errorcluster, "CompressorDevRef"=w69:T18)  [unwired: 9 in]
  n102 = call <vilib>:"WPI_JoystickGetValues.vi"("JoystickDevRef"=w105) -> ("Buttons"=w100:bool[], "Axes"=w101:dbl[])  [unwired: 6 in, 3 out]
  n103 = call <vilib>:"WPI_CompressorGetEnableState.vi"("error in (no error)"=w70, "CompressorDevRef"=w69) -> ("Compressor Running"=→"Compressor Running":bool, "Enabled"=→"Enabled":bool)  [unwired: 6 in, 2 out]
  n104 = Index Array(array=w101) -> ()  [unwired: 2 in, 2 out]
  n105 = call-poly <vilib>:"NT Write Value.vi"("Numeric Array"=w101, "Name"="Joystick 0/Axes") -> ()  [unwired: 9 in, 1 out]
  n106 = call-poly <vilib>:"NT Write Value.vi"("Boolean Array"=w100, "Name"="Joystick 0/Buttons") -> ()  [unwired: 9 in, 1 out]
  n107 = disable-structure shown="Disabled" {
    frame Disabled {
      n108 = case shown="False" FALSE {
        tunnel: 0 -> [w250 w253]
        tunnel: [w250 w251] -> w244
        frame False {
        }
        frame True {
          n109 = Add(x=w253, y=1) -> (x+y=w251:i32)
        }
      }
      n110 = Divide(x=w244, y=2) -> (x/y=w243:dbl)
      n111 = Equal?(x=w243, y=0.0) -> (x = y?=w240:bool)
      n112 = Select(t=WPI_SolenoidValue."Reverse" ("Value"), s=w240, f=WPI_SolenoidValue."Forward" ("Value")) -> (s? t:f=w246:T12)
      n113 = call <vilib>:"WPI_SolenoidRefNum Registry Get.vi"("refnum name"="ThirdStage0") -> ("error out"=w248:errorcluster, "SolenoidDevRef"=w247:T13)  [unwired: 9 in]
      n114 = call-poly <vilib>:"WPI_SolenoidSet.vi"("error in (no error)"=w248, "Value"=w246, "SolenoidDevRef"=w247) -> ()  [unwired: 7 in, 2 out]
    }
    frame Enabled {
    }
  }
